vi "CTRE_ServoBlock_TankStraightImu.vi"(10 "Timeout":dbl, 11 "Tank Straight IMU":T11 {"PigeonIMU"."Type" items=["CAN"=352321536, "TalonSRX"=33554432]}) -> (3 "Tank Drivetrain":T1={"Left Gearbox"={"SmartMotorController 1"={"DeviceStatus"={"status"=FALSE, "code"=0, "source"=""}, "Type"=enum."PWM", "PWM"={"PWM Channel"=enum."PWM 1", "DeadBand"={"Name"="", "maxPositivePwm"=0, "minPositivePwm"=0, "centerPwm"=0, "maxNegativePwm"=0, "minNegativePwm"=0, "angularRange"=0}}, "CAN"={"Device Number"=0, "SetOutput VI Ref"=variant(enum8{"Percent VBus", "Current", "Speed", "Position", "Voltage"} enum."Percent VBus"), "GetOutput VI Ref"=variant(refnum<k1> refnum), "Enable VI Ref"=variant(dbl 12.0), "Disable VI Ref"=variant(enum8{"Percent VBus", "Speed", "Position", "Slave", "Unchanged / Invalid", "Voltage Compensation", "Current", "Motion Profile"} enum."Percent VBus"), "Data"=variant}, "Invert"=FALSE}, "Invert"=FALSE}, "Right Gearbox"={"SmartMotorController 1"={"DeviceStatus"={"status"=FALSE, "code"=0, "source"=""}, "Type"=enum."PWM", "PWM"={"PWM Channel"=enum."PWM 1", "DeadBand"={"Name"="", "maxPositivePwm"=0, "minPositivePwm"=0, "centerPwm"=0, "maxNegativePwm"=0, "minNegativePwm"=0, "angularRange"=0}}, "CAN"={"Device Number"=0, "SetOutput VI Ref"=variant(enum8{"Percent VBus", "Current", "Speed", "Position", "Voltage"} enum."Percent VBus"), "GetOutput VI Ref"=variant(refnum<k1> refnum), "Enable VI Ref"=variant(dbl 12.0), "Disable VI Ref"=variant(enum8{"Percent VBus", "Speed", "Position", "Slave", "Unchanged / Invalid", "Voltage Compensation", "Current", "Motion Profile"} enum."Percent VBus"), "Data"=variant}, "Invert"=FALSE}, "Invert"=FALSE}})   [LabVIEW 2016]
uses:
  <vilib>/Rock Robotics/WPI/ThirdParty/CanMotor/CTRLib-LV-TalonSRX/Framework/Tank.ctl
  <vilib>/Rock Robotics/WPI/ThirdParty/CanMotor/CTRLib-LV-TalonSRX/Framework/Gearbox.ctl
  <vilib>/Rock Robotics/WPI/MotorControl/WPI_MotorControlDeviceRef.ctl
  <vilib>/Rock Robotics/WPI/MotorControl/WPI_MotorControlType.ctl
  <vilib>/Rock Robotics/SystemInterfaces/DIO/FPGA_DIOPWMChannel.ctl
  <vilib>/Rock Robotics/WPI/PWM/WPI_PWMDeadband.ctl
  <vilib>/Rock Robotics/WPI/ThirdParty/Sensors/Pigeon IMU/CTRE_PigeonIMU_DeviceRef.ctl
  <vilib>/Rock Robotics/WPI/ThirdParty/Sensors/Pigeon IMU/CTRE_PigeonIMU_ConnectionType.ctl
  <vilib>/Rock Robotics/WPI/ThirdParty/CanMotor/CTRLib-LV-TalonSRX/CTRE_CANTalonSRX_ControlMode.ctl
  <vilib>/Rock Robotics/WPI/ThirdParty/CanMotor/CTRLib-LV-TalonSRX/Framework/ServoParams.ctl
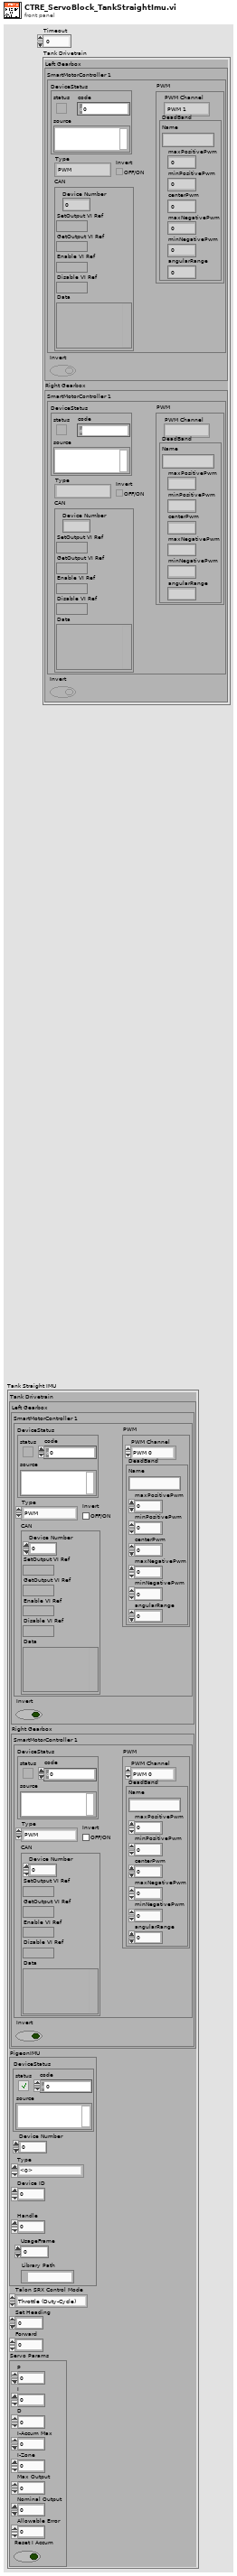
[diagram p1: front panel]
types:
  T1 = typedef "Tank.ctl" = cluster{"Left Gearbox":T2, "Right Gearbox":T2}
  T2 = typedef "Gearbox.ctl" = cluster{"SmartMotorController 1":T3, "Invert":bool}
  T3 = typedef "WPI_MotorControlDeviceRef.ctl" = cluster{"DeviceStatus":errorcluster, "Type":T4, "PWM":cluster{"PWM Channel":T5, "DeadBand":T6}, "CAN":cluster{"Device Number":u8, "SetOutput VI Ref":variant, "GetOutput VI Ref":variant, "Enable VI Ref":variant, "Disable VI Ref":variant, "Data":variant}, "Invert":bool}
  T4 = typedef "WPI_MotorControlType.ctl" = enum16{"PWM", "CAN"}
  T5 = typedef "FPGA_DIOPWMChannel.ctl" = enum8{"PWM 0", "PWM 1", "PWM 2", "PWM 3", "PWM 4", "PWM 5", "PWM 6", "PWM 7", "PWM 8", "PWM 9", "PWM MXP 0", "PWM MXP 1", "PWM MXP 2", "PWM MXP 3", "PWM MXP 4", "PWM MXP 5", "PWM MXP 6", "PWM MXP 7", "PWM MXP 8", "PWM MXP 9", "Invalid"}
  T6 = typedef "WPI_PWMDeadband.ctl" = cluster{"Name":string, "maxPositivePwm":i32, "minPositivePwm":i32, "centerPwm":i32, "maxNegativePwm":i32, "minNegativePwm":i32, "angularRange":u16}
  T7 = typedef "CTRE_PigeonIMU_DeviceRef.ctl" = cluster{"DeviceStatus":errorcluster, "Device Number":u8, "Type":T8, "Device ID":u32, "Handle":u64, "UsageFrame":u32, "Library Path":path}
  T8 = typedef "CTRE_PigeonIMU_ConnectionType.ctl" = u32
  T9 = typedef "CTRE_CANTalonSRX_ControlMode.ctl" = enum16{"Throttle (Duty-Cycle)", "Position Closed-Loop", "Velocity Closed-Loop", "Current Closed-Loop", "Voltage Compensation", "Slave Follower", "Motion Profile", "Motion Magic"}
  T10 = typedef "ServoParams.ctl" = cluster{"P":dbl, "I":dbl, "D":dbl, "I-Accum Max":dbl, "I-Zone":dbl, "Max Output":dbl, "Nominal Output":dbl, "Allowable Error":dbl, "Reset I Accum":bool}
  T11 = cluster{"Tank Drivetrain":T1, "PigeonIMU":T7, "Talon SRX Control Mode":T9, "Set Heading":dbl, "Forward":dbl, "Servo Params":T10}
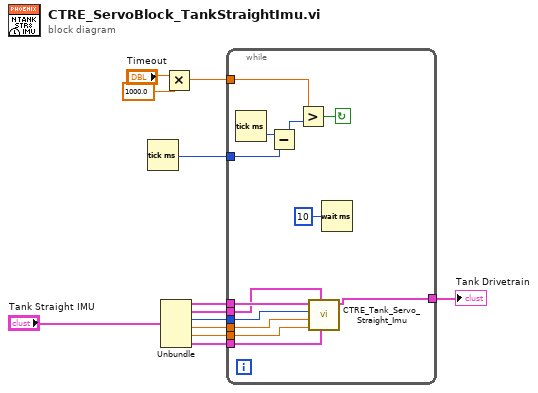
[diagram p0: block diagram]
diagram:
  n1 = Tick Count (ms)() -> (millisecond timer value=w6:u32)
  n2 = Unbundle("Tank Straight IMU") -> ("Tank Drivetrain"=w12:T1, "PigeonIMU"=w11:T7, "Talon SRX Control Mode"=w10:T9, "Set Heading"=w9:dbl, "Forward"=w8:dbl, "Servo Params"=w7:T10)
  n3 = Multiply(x="Timeout", y=1000.0) -> (x*y=w3:dbl)
  n4 = while {
    tunnel: w12 -> [w25]
    tunnel: w11 -> [w24]
    tunnel: w10 -> [w23]
    tunnel: w9 -> [w22]
    tunnel: w8 -> [w21]
    tunnel: w7 -> [w20]
    tunnel: w6 -> [w18]
    tunnel: w3 -> [w16]
    tunnel: [w13] -> w2
    stop <- w15 continue-if-true
    n5 = Tick Count (ms)() -> (millisecond timer value=w19:u32)
    n6 = Subtract(x=w19, y=w18) -> (x-y=w17:u32)
    n7 = Greater?(x=w16, y=w17) -> (0:w15:bool)
    n8 = call <vilib>:"CTRE_Tank_Servo_Straight_Imu.vi"("Servo Params"=w20, "PigeonIMU"=w24, "Forward"=w21, "Set Heading"=w22, "Talon SRX Control Mode"=w23, "Tank Drivetrain"=w25) -> ("Tank Drivetrain"=w13:T1)  [unwired: 3 in, 2 out]
    n9 = Wait (ms)(milliseconds to wait=u32 10) -> ()  [unwired: 1 out]
  }
  "Tank Drivetrain" <- w2
